vi "Overtime.vi"   [LabVIEW 2020]
uses:
  <vilib>/Rock Robotics/WPI/Solenoid/WPI_SolenoidValue.ctl
  <vilib>/Rock Robotics/WPI/Utilities/WPI_GetSetVariantRefNum.vi
  <vilib>/Rock Robotics/WPI/Solenoid/WPI_SolenoidSetEnum.vi
types:
  T1 = typedef "WPI_SolenoidValue.ctl" = enum16{"Off", "On", "Forward", "Reverse"}
  T2 = typedef "WPI_JoystickDevRef.ctl" = cluster{"Device":T3}
  T3 = typedef "WPI_JoystickDeviceEnum.ctl" = enum16{"USB 0", "USB 1", "USB 2", "USB 3", "USB 4", "USB 5"}
  T4 = typedef "WPI_SolenoidDevRef.ctl" = cluster{"DevStatus":errorcluster, "Pneumatics Control Module":u8, "Forward Solenoid Channel":T5, "Reverse Solenoid Channel":T5}
  T5 = typedef "WPI_SolenoidChannel.ctl" = enum8{"Solenoid 0", "Solenoid 1", "Solenoid 2", "Solenoid 3", "Solenoid 4", "Solenoid 5", "Solenoid 6", "Solenoid 7", "Solenoid 8", "Solenoid 9", "Solenoid 10", "Solenoid 11", "Solenoid 12", "Solenoid 13", "Solenoid 14", "Solenoid 15", "Invalid"}
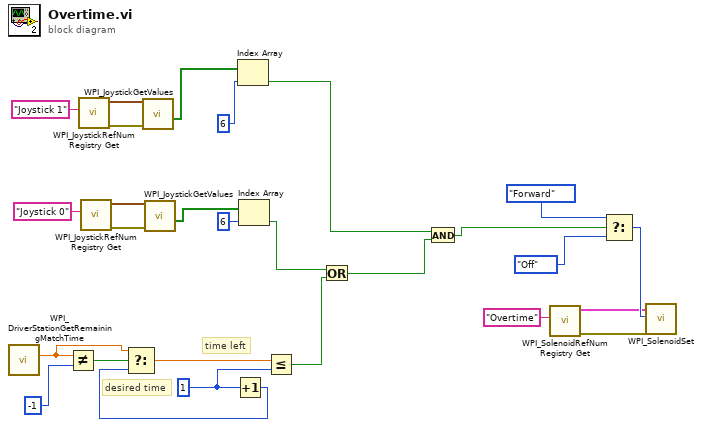
[diagram p0: block diagram]
diagram:
  w21 = 1
  # "desired time"
  # "time left"
  n1 = call <vilib>:"WPI_DriverStationGetRemainingMatchTime.vi"() -> ("Match Time(s)"=w23:sgl)  [unwired: 10 in, 1 out]
  n2 = Not Equal?(x=w23, y=-1) -> (x != y?=w24:bool)
  n3 = call <vilib>:"WPI_JoystickRefNum Registry Get.vi"("refnum name"="Joystick 1") -> ("error out"=w18:errorcluster, "JoystickDevRef"=w19:T2)  [unwired: 9 in]
  n4 = call <vilib>:"WPI_JoystickRefNum Registry Get.vi"("refnum name"="Joystick 0") -> ("error out"=w15:errorcluster, "JoystickDevRef"=w16:T2)  [unwired: 9 in]
  n5 = call <vilib>:"WPI_JoystickGetValues.vi"("error in (no error)"=w18, "JoystickDevRef"=w19) -> ("Buttons"=w13:bool[])  [unwired: 5 in, 4 out]
  n6 = call <vilib>:"WPI_JoystickGetValues.vi"("error in (no error)"=w15, "JoystickDevRef"=w16) -> ("Buttons"=w12:bool[])  [unwired: 5 in, 4 out]
  n7 = Increment(x=w21) -> (x+1=w20:i32)
  n8 = Select(t=w23, s=w24, f=w20) -> (s? t:f=w22:sgl)
  n9 = Index Array(array=w13, index=6) -> (element=w8:bool)
  n10 = Index Array(array=w12, index=6) -> (element=w9:bool)
  n11 = Less Or Equal?(x=w22, y=w21) -> (x <= y?=w27:bool)
  n12 = Or(x=w9, y=w27) -> (x .or. y?=w26:bool)
  n13 = And(x=w8, y=w26) -> (x .and. y?=w6:bool)
  n14 = call <vilib>:"WPI_SolenoidRefNum Registry Get.vi"("refnum name"="Overtime") -> ("error out"=w1:errorcluster, "SolenoidDevRef"=w3:T4)  [unwired: 9 in]
  n15 = Select(t=WPI_SolenoidValue."Forward" ("Value"), s=w6, f=WPI_SolenoidValue."Off" ("Value")) -> (s? t:f=w4:T1)
  n16 = call-poly <vilib>:"WPI_SolenoidSet.vi"("error in (no error)"=w1, "Value"=w4, "SolenoidDevRef"=w3) -> ()  [unwired: 7 in, 2 out]
